vi "실습 7-3.vi"() -> ()   [LabVIEW 2014]
uses:
  winmm.dll
panel:
  out "Success?":bool
  in  "경로":path
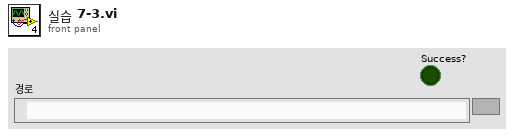
[diagram p1: front panel]
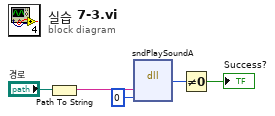
[diagram p0: block diagram]
diagram:
  n1 = Path To String(path="경로") -> (string=w4:string)
  n2 = dll-call lib="winmm.dll" fn="sndPlaySoundA"("SoundFile"=w4, "options"=u32 0) -> ("반환 타입"=w2:i32)  [unwired: 5 in, 2 out]
  n3 = Not Equal To 0?(x=w2) -> (x != 0?=→"Success?":bool)
